vi "Test_PublicationLocked_OwnerUnlocks_OK.vi"(8 "error in (no error)":errorcluster, 11 "TestMediator In":refnum<class "TestMediator.lvclass">) -> (0 "error out":errorcluster, 3 "TestMediator Out":refnum<class "TestMediator.lvclass">)   [LabVIEW 2015, in "TestMediator.lvclass"]
uses:
  TestMediator.lvclass
  Mediator/Mediator.lvclass
  IMediator/PublishRequest/PublishRequest.lvclass/PublishRequest.ctl
  Transport/QueueTransport/QueueTransport.lvclass/QueueTransport.ctl
  SubscriptionPolicy/BasicSubscription/BasicSubscription.lvclass/BasicSubscription.ctl
  IMediator/SubscriptionRequest/SubscriptionRequest.lvclass/SubscriptionRequest.ctl
  IMediator/IMediator Messages/Lock Publication Msg/Lock Publication Msg.lvclass/Lock Publication Msg.ctl
  <vilib>/ActorFramework/Message Enqueuer/Message Enqueuer.lvclass/Message Enqueuer.ctl
  IMediator/IMediator Messages/Unlock Publication Msg/Unlock Publication Msg.lvclass/Unlock Publication Msg.ctl
  IMediator/IMediator Messages/Publish Msg/Publish Msg.lvclass/Publish Msg.ctl
  IMediator/IMediator Messages/Subscribe Msg/Subscribe Msg.lvclass/Subscribe Msg.ctl
  <vilib>/ActorFramework/Message Enqueuer/Enqueue.vi
  <vilib>/Utility/error.llb/Error Cluster From Error Code.vi
  <vilib>/ActorFramework/Message Priority Queue/Priority Enqueue.vi
  SubscriptionPolicy/BasicSubscription/BasicSubscription.lvclass
  Transport/QueueTransport/QueueTransport.lvclass
  IMediator/SubscriptionRequest/SubscriptionRequest.lvclass
  IMediator/IPublicationPolicy/IPublicationPolicy.lvclass
  IMediator/ITransport/ITransport.lvclass
  IMediator/IMediator Messages/Lock Publication Msg/Lock Publication Msg.lvclass
  IMediator/IMediator Messages/Unlock Publication Msg/Unlock Publication Msg.lvclass
  IMediator/PublishRequest/PublishRequest.lvclass
  IMediator/IMediator Messages/Publish Msg/Publish Msg.lvclass
  IMediator/IMediator Messages/Subscribe Msg/Subscribe Msg.lvclass
  <vilib>/ActorFramework/Stop Msg/Stop Msg.lvclass
  <vilib>/addons/_JKI Toolkits/VI Tester/TestCase.llb/TestCase.lvclass
  <vilib>/ActorFramework/Actor/Actor.lvclass
  IMediator/ISubscriptionPolicy/ISubscriptionPolicy.lvclass
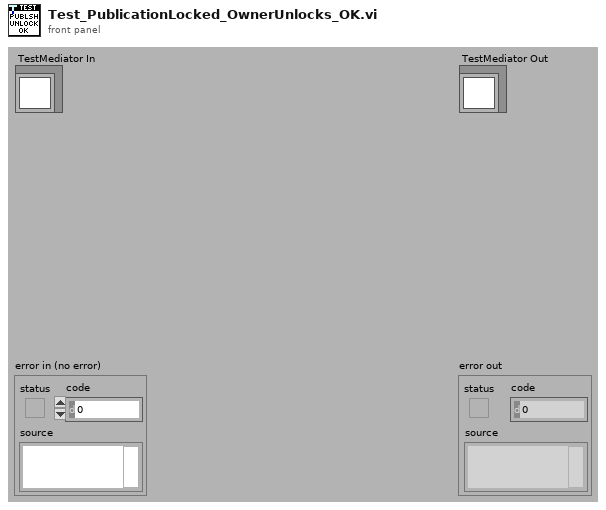
[diagram p1: front panel]
types:
  T1 = typedef "IMediator.lvlib/ISubscriptionPolicy.lvclass/ISubscriptionPolicy Reference.ctl" = refnum<data-value>
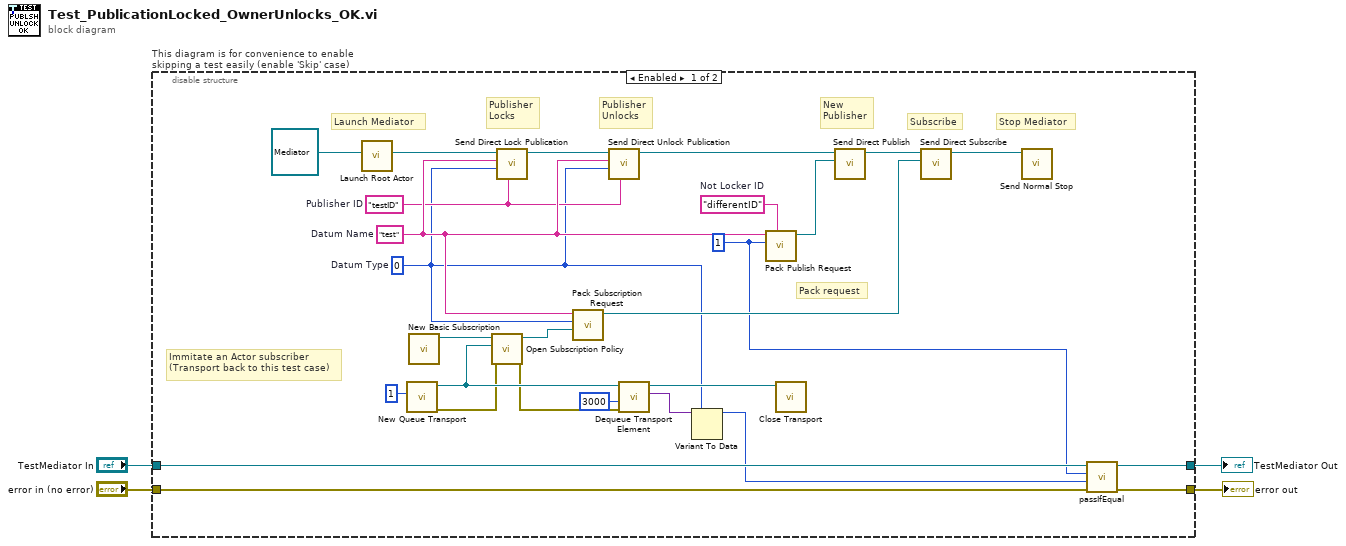
[diagram p0: block diagram]
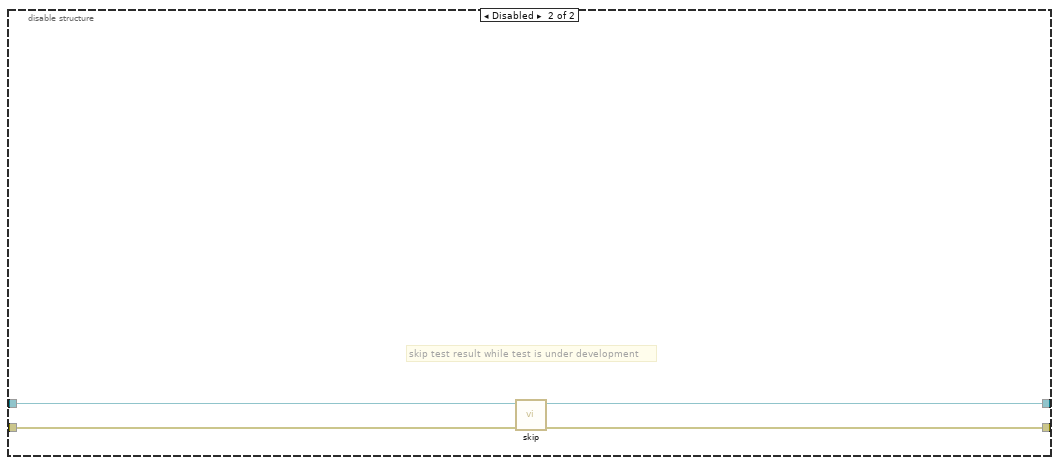
[diagram p2: hidden frame]
diagram:
  n1 = disable-structure "This diagram is for convenience to enable skipping a test easily (enable 'Skip' case)" shown="Enabled" {
    disable-tunnel: "TestMediator In" -> [w31 w35]
    disable-tunnel: [w30 w33] -> w1
    disable-tunnel: [w29 w34] -> w3
    disable-tunnel: "error in (no error)" -> [w28 w32]
    frame Enabled {
      w12 = "differentID"  # Not Locker ID
      w9 = "testID"  # Publisher ID
      w6 = 0  # Datum Type
      w10 = "test"  # Datum Name
      w5 = 1
      # "Publisher\nUnlocks"
      # "Immitate an Actor subscriber\n(Transport back to this test case)"
      # "Pack request"
      # "Publisher\nLocks"
      # "Launch Mediator"
      # "Stop Mediator"
      # "Subscribe"
      # "New\nPublisher"
      n2 = call <vilib>:"Launch Root Actor.vi"("Actor"=refnum<class "Mediator.lvclass"> refnum ("Mediator.lvlib:Mediator.lvclass")) -> ("Actor's Enqueuer"=w26:refnum<class "Message Enqueuer.lvclass">)  [unwired: 9 in, 1 out]
      n3 = call "New Queue Transport.vi"("Max Queue Size (-1)"=1) -> ("error out"=w20:errorcluster, "QueueTransport"=w22:refnum<class "QueueTransport.lvclass">)  [unwired: 9 in]
      n4 = call "New Basic Subscription.vi"() -> ("BasicSubscription Out"=w16:refnum<class "BasicSubscription.lvclass">)  [unwired: 11 in]
      n5 = call "Open Subscription Policy.vi"("error in (no error)"=w20, "Transport"=w22, "SubscriptionPolicy"=w16) -> ("error out"=w19:errorcluster, "Subscription Policy"=w15:T1)  [unwired: 7 in]
      n6 = call "Send Direct Lock Publication.vi"("Publisher ID"=w9, "Datum Type"=w6, "Datum Name"=w10, "Mediator Enqeuer"=w26) -> ("Mediator Enqueuer out"=w13:refnum<class "Message Enqueuer.lvclass">)  [unwired: 6 in, 1 out]
      n7 = call "Pack Subscription Request.vi"("Subscription Policy"=w15, "Type"=w6, "Datum Name"=w10) -> ("SubscriptionRequest"=w25:refnum<class "SubscriptionRequest.lvclass">)  [unwired: 8 in]
      n8 = call "Send Direct Unlock Publication.vi"("Publisher ID"=w9, "Datum Type"=w6, "Datum Name"=w10, "Mediator Enqeuer"=w13) -> ("Mediator Enqueuer out"=w11:refnum<class "Message Enqueuer.lvclass">)  [unwired: 6 in, 1 out]
      n9 = call "Dequeue Transport Element.vi"("error in (no error)"=w19, "Timeout In ms (-1)"=3000, "QueueTransport in"=w22) -> ("Data"=w8:variant, "QueueTransport out"=w17:refnum<class "QueueTransport.lvclass">)  [unwired: 5 in, 2 out]
      n10 = Variant To Data(type=w6, Variant=w8) -> (data=w7:i32)  [unwired: 1 in, 1 out]
      n11 = call "Pack Publish Request.vi"("Publisher ID"=w12, "Data to Publish"=w5, "Datum Name"=w10) -> ("PublishRequest"=w14:refnum<class "PublishRequest.lvclass">)  [unwired: 8 in]
      n12 = call-dynamic "Close Transport.vi"("QueueTransport in"=w17) -> ()  [unwired: 10 in, 1 out]
      n13 = call "Send Direct Publish.vi"("PublishRequest"=w14, "Mediator Enqeuer"=w11) -> ("Mediator Enqueuer out"=w24:refnum<class "Message Enqueuer.lvclass">)  [unwired: 8 in, 1 out]
      n14 = call "Send Direct Subscribe.vi"("Subscription Request"=w25, "Message Enqueuer"=w24) -> ("Message Enqueuer out"=w18:refnum<class "Message Enqueuer.lvclass">)  [unwired: 8 in, 1 out]
      n15 = call <vilib>:"Send Normal Stop.vi"("Message Enqueuer"=w18) -> ()  [unwired: 10 in, 1 out]
      n16 = call-dynamic "passIfEqual.vi"("error in (no error)"=w28, "y"=w7, "x"=w5, "TestCase in"=w31) -> ("error out"=w29:errorcluster, "TestCase out"=w30:refnum<class "TestMediator.lvclass">)  [unwired: 6 in]
    }
    frame Disabled {
      # "skip test result while test is under development"
      n17 = call <vilib>:"skip.vi"("error in (no error)"=w32, "TestCase in"=w35) -> ("error out"=w34:errorcluster, "TestCase out"=w33:refnum<class "TestMediator.lvclass">)  [unwired: 8 in]
    }
  }
  "error out" <- w3
  "TestMediator Out" <- w1
